vi "Basic Dual RT Setup.vi"(8 "error in (no error)":errorcluster, 11 "1553 Test in":refnum<class "1553 Test.lvclass">) -> (0 "error out":errorcluster, 3 "1553 Test out":refnum<class "1553 Test.lvclass">)   [LabVIEW 2016, in "1553 Test.lvclass"]
uses:
  1553 Test.lvclass
  1553 Component/1553 Component.lvclass
  Remote Terminal/Remote Terminal.lvclass
  Remote Terminal/TypeDefs/RT Configuration.ctl
  1553 SubComponent/TypeDefs/Scaling Information.ctl
  1553 SubComponent/TypeDefs/Parameter Table Data.ctl
  Remote Terminal/TypeDefs/Command Type.ctl
  Remote Terminal/TypeDefs/Command Configuration.ctl
  Remote Terminal/TypeDefs/RT Timetag Configuration.ctl
  Remote Terminal/TypeDefs/Mode Code 17 Sync Configuration.ctl
  Remote Terminal/TypeDefs/RT-RT Timeout.ctl
  D:/R&D/cRIO 1553 2016/Windows/1553 SubComponent/1553 SubComponent.lvclass
  Dependencies/FPGA Interface/FPGA Interface.lvclass
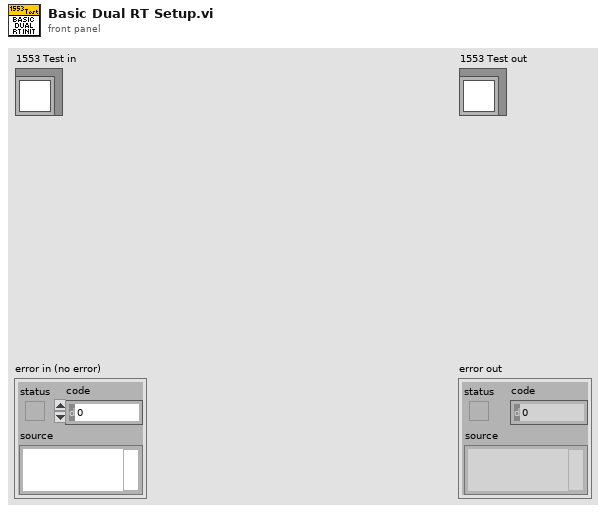
[diagram p1: front panel]
types:
  T1 = typedef "BCI-1553 API.lvlib/Remote Terminal.lvclass/Command Configuration.ctl" = cluster{"Command Type":T2, "Mode Code ID (1-32)":u16, "SubAddress (1-30)":u16, "Word Count (1-32)":u16, "Illegal Command":bool, "Broadcast":bool, "Data":u16[], "Data Fields":T3[]}
  T2 = typedef "BCI-1553 API.lvlib/Remote Terminal.lvclass/Command Type.ctl" = enum16{"Transmit", "Receive", "Mode Code Tx", "Mode Code Rx"}
  T3 = typedef "BCI-1553 API.lvlib/1553 SubComponent.lvclass/Parameter Table Data.ctl" = cluster{"Parameter Name":string, "Base Word":u16, "Address":u16, "Value":u64, "Mask":u16[], "Scaling Info":T4}
  T4 = typedef "BCI-1553 API.lvlib/1553 SubComponent.lvclass/Scaling Information.ctl" = cluster{"Bit Offset":i32, "Bit Count":i32, "LSB Resolution":dbl, "2's Complement":bool, "Big Endian":bool, "Sign Bit":bool}
  T5 = typedef "BCI-1553 API.lvlib/Remote Terminal.lvclass/RT Configuration.ctl" = cluster{"RT-RT Timeout":T6, "Inhibit Bus A":bool, "Inhibit Bus B":bool, "Broadcast CMD Invalid":bool, "UnDef MCs Invalid":bool, "Notice 2 Data Storage":bool, "SMCP":bool, "Temp RX Buffer":bool, "Alt BIT Enable":bool, "Auto Bus Shutdown":bool, "MC 16 SR Reset":bool, "MC 17 Sync":T7, "MC 8 Reset":bool, "Remote Terminal Timetag Config":T8}
  T6 = typedef "BCI-1553 API.lvlib/Remote Terminal.lvclass/RT-RT Timeout.ctl" = enum16{"57us", "62us", "100us", "180us"}
  T7 = typedef "BCI-1553 API.lvlib/Remote Terminal.lvclass/Mode Code 17 Sync Configuration.ctl" = enum16{"Sync if Bit 0 = 1", "Sync if Bit 0 = 0", "Sync Unconditionally"}
  T8 = typedef "BCI-1553 API.lvlib/Remote Terminal.lvclass/RT Timetag Configuration.ctl" = enum16{"Disabled", "2us", "4us", "8us", "16us", "32us", "64us"}
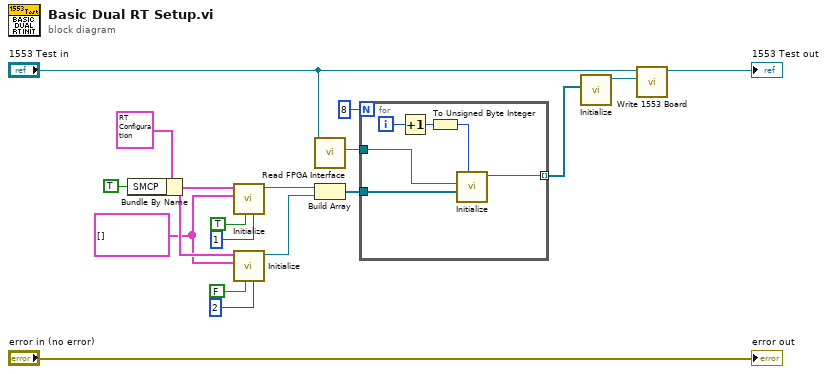
[diagram p0: block diagram]
diagram:
  w4 = T1[] [] ("Commands")
  n1 = Bundle By Name(cluster=T5 {"RT-RT Timeout"=enum."57us", "Inhibit Bus A"=FALSE, "Inhibit Bus B"=FALSE, "Broadcast CMD Invalid"=FALSE, "UnDef MCs Invalid"=FALSE, "Notice 2 Data Storage"=FALSE, "SMCP"=FALSE, "Temp RX Buffer"=FALSE, "Alt BIT Enable"=FALSE, "Auto Bus Shutdown"=FALSE, "MC 16 SR Reset"=FALSE, "MC 17 Sync"=enum."Sync if Bit 0 = 1", "MC 8 Reset"=FALSE, "Remote Terminal Timetag Config"=enum."Disabled"} ("RT Configuration"), "SMCP"=TRUE) -> (w14:T5)
  n2 = call "Initialize.vi"("Terminal Address"=u8 1 ("RT Address (0-30)"), "RT 1?"=TRUE, "RT Commands"=w4, "RT Configuration"=w14) -> ("Remote Terminal out"=w13:refnum<class "Remote Terminal.lvclass">)  [unwired: 6 in, 1 out]
  n3 = call "Initialize.vi"("Terminal Address"=u8 2 ("RT Address (0-30)"), "RT 1?"=FALSE, "RT Commands"=w4, "RT Configuration"=w14) -> ("Remote Terminal out"=w12:refnum<class "Remote Terminal.lvclass">)  [unwired: 6 in, 1 out]
  n4 = call-dynamic "Read FPGA Interface.vi"("1553 Test in"="1553 Test in") -> ("FPGA Interface"=w10:refnum<class "FPGA Interface.lvclass">)  [unwired: 8 in, 2 out]
  n5 = Build Array(w13, w12) -> (w11:refnum<class "Remote Terminal.lvclass">[])
  n6 = for {
    N: 8 -> [_]
    tunnel: [w22] -> w16 mode=indexing
    tunnel: w11 -> [w21]
    tunnel: w10 -> [w20]
    i -> [w24]
    n7 = Increment(x=w24) -> (x+1=w19:i32)
    n8 = To Unsigned Byte Integer(number=w19) -> (unsigned 8bit integer=w23:u8)
    n9 = call "Initialize.vi"("Component ID (1-8)"=w23, "SubComponents"=w21, "FPGA Interface"=w20) -> ("1553 Component out"=w22:refnum<class "1553 Component.lvclass">)  [unwired: 7 in, 1 out]
  }
  n10 = call "Initialize.vi"("Components"=w16) -> ("1553 Board out"=w17:refnum<class "1553 Board.lvclass">)  [unwired: 9 in, 1 out]
  n11 = call-dynamic "Write 1553 Board.vi"("1553 Board"=w17, "1553 Test in"="1553 Test in") -> ("1553 Test out"=→"1553 Test out":refnum<class "1553 Test.lvclass">)  [unwired: 8 in, 1 out]
  "error out" <- "error in (no error)"
